vi "Start Main Program.vi"(8 "error in (no error)":errorcluster, 11 "VISA resource name":refnum<visa-resource-name>) -> (0 "error out":errorcluster, 3 "VISA resource name out":refnum<visa-resource-name>)   [LabVIEW 2017, in "JY-SPEX-TRIAX.lvlib"]
doc: "Starts the main spectrometer controller program (loaded in firmware)."
uses:
  JY-SPEX-TRIAX.lvlib
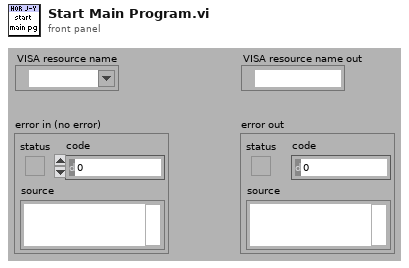
[diagram p1: front panel]
types:
  T1 = typedef "Semaphore RefNum" = refnum<k1>
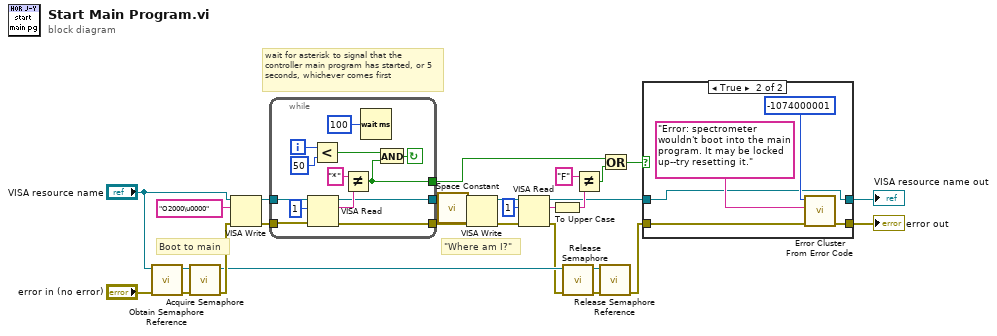
[diagram p0: block diagram]
diagram:
  # "\"Where am I?\""
  # "Boot to main"
  # "wait for asterisk to signal that the controller main program has started, or 5 seconds, whichever comes first"
  n1 = call <vilib>:"Obtain Semaphore Reference.vi"("error in (no error)"="error in (no error)", "name (unnamed)"="VISA resource name") -> ("error out"=w11:errorcluster, "semaphore"=w10:T1)  [unwired: 1 in, 3 out]
  n2 = call <vilib>:"Acquire Semaphore.vi"("error in (no error)"=w11, "semaphore"=w10) -> ("error out"=w7:errorcluster, "semaphore out"=w4:T1)  [unwired: 1 in, 3 out]
  n3 = VISA Write(VISA resource name="VISA resource name", write buffer="O2000\u0000", error in (no error)=w7) -> (VISA resource name out=w14:refnum<visa-resource-name>, error out=w13:errorcluster)  [unwired: 1 out]
  n4 = while {
    tunnel: [w38] -> w27
    tunnel: [w37] -> w26
    tunnel: [w29] -> w18
    tunnel: w14 -> [w35]
    tunnel: w13 -> [w36]
    i -> [w33]
    stop <- w30 continue-if-true
    n5 = VISA Read(VISA resource name=w35, byte count=u32 1, error in (no error)=w36) -> (VISA resource name out=w38:refnum<visa-resource-name>, read buffer=w40:string, error out=w37:errorcluster)  [unwired: 1 out]
    n6 = Less?(x=w33, y=50) -> (x < y?=w31:bool)
    n7 = Not Equal?(x="*", y=w40) -> (x != y?=w29:bool)
    n8 = Wait (ms)(milliseconds to wait=u32 100) -> ()  [unwired: 1 out]
    n9 = And(x=w31, y=w29) -> (x .and. y?=w30:bool)
  }
  n10 = call <vilib>:"Space Constant.vi"() -> ("String"=w25:string)
  n11 = VISA Write(VISA resource name=w27, write buffer=w25, error in (no error)=w26) -> (VISA resource name out=w23:refnum<visa-resource-name>, error out=w24:errorcluster)  [unwired: 1 out]
  n12 = VISA Read(VISA resource name=w23, byte count=u32 1, error in (no error)=w24) -> (VISA resource name out=w15:refnum<visa-resource-name>, read buffer=w21:string, error out=w3:errorcluster)  [unwired: 1 out]
  n13 = To Upper Case(1:w21) -> (0:w20:string)
  n14 = call <vilib>:"Release Semaphore.vi"("error in (no error)"=w3, "semaphore"=w4) -> ("error out"=w6:errorcluster, "semaphore out"=w5:T1)  [unwired: 4 out]
  n15 = Not Equal?(x="F", y=w20) -> (x != y?=w17:bool)
  n16 = call <vilib>:"Release Semaphore Reference.vi"("error in (no error)"=w6, "semaphore"=w5) -> ("error out"=w2:errorcluster)  [unwired: 9 out]
  n17 = Or(x=w18, y=w17) -> (x .or. y?=w16:bool)
  n18 = case shown="True" w16 {
    tunnel: w2 -> [w42 w46]
    tunnel: w15 -> [w43 w44]
    tunnel: [w43 w44] -> w12
    tunnel: [w42 w45] -> w1
    frame False {
    }
    frame True {
      n19 = call <vilib>:"Error Cluster From Error Code.vi"("error in (no error)"=w46, "error message (\"\")"="Error: spectrometer wouldn't boot into the main program. It may be locked up--try resetting it." ("error message (\"\")"), "error code (0)"=-1074000001) -> ("error out"=w45:errorcluster)  [unwired: 1 in, 5 out]
    }
  }
  "VISA resource name out" <- w12
  "error out" <- w1
